vi "Value_Selection_in_Table_GUI.vi"(9 "Column Headers":string[](array[string]), 11 "SELECTION TABLE - Click on values to keep":string[][](table)) -> (2 "Coordinate Array":i32[][](array[numeric]))   [LabVIEW 2020]
uses:
  <vilib>/Utility/miscctls.llb/LVRowAndColumnTypeDef.ctl
  405f9b96-5d72-4015-90c1-6a1ff41fe83b.vi
panel:
  in  "RESET":bool
  in  "DONE":bool
  # "How to use :\n1. The green values are kept\n2. Click the ECS cell if you want to keep the ECS Value.\n2. Reclick the ECS cell if you want to revert to preset value"
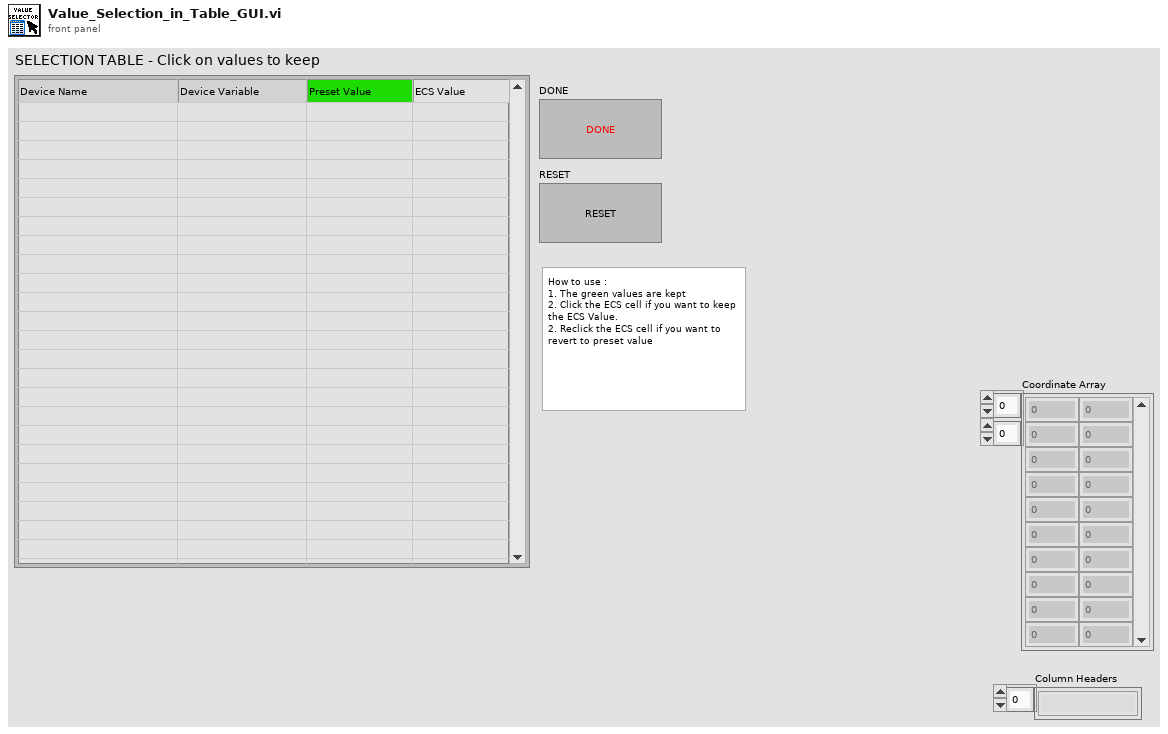
[diagram p1: front panel]
types:
  T1 = typedef "LVRowAndColumnTypeDef.ctl" = cluster{"Row":i32, "Column":i32}
  T2 = typedef "LVPoint32TypeDef.ctl" = cluster{"Horizontal":i32, "Vertical":i32}
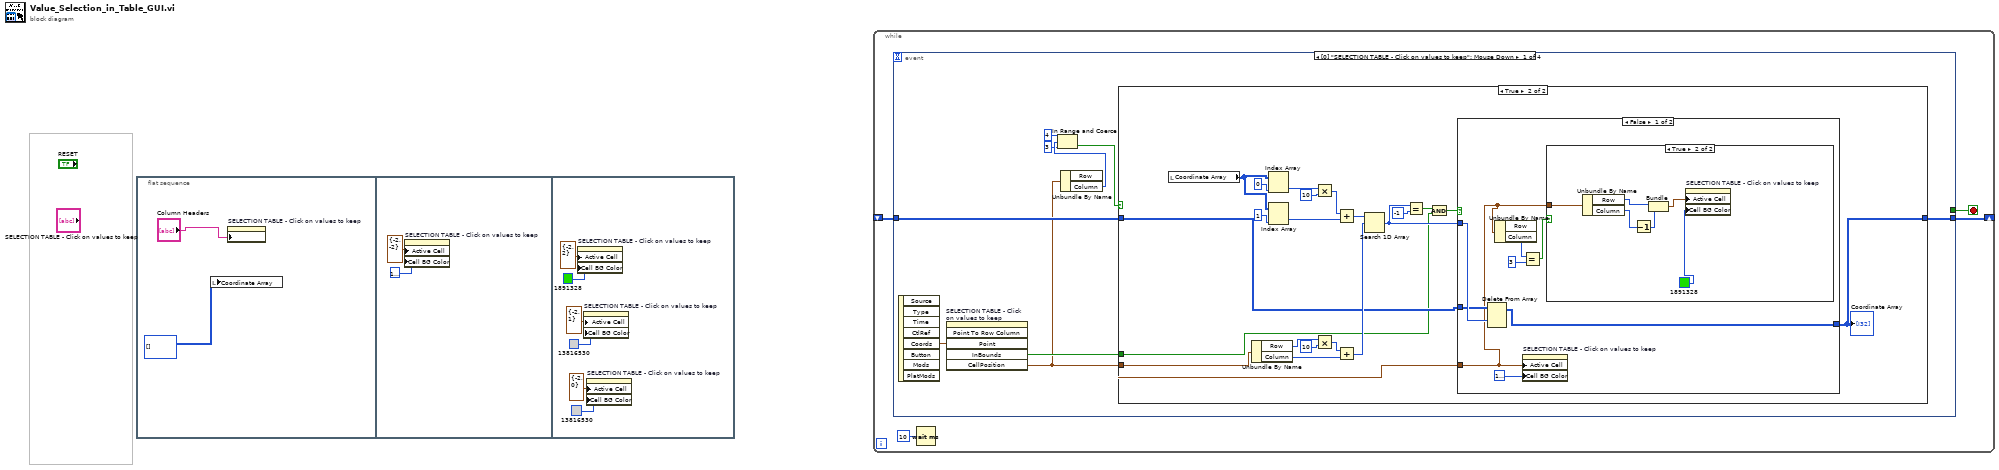
[diagram p0: block diagram]
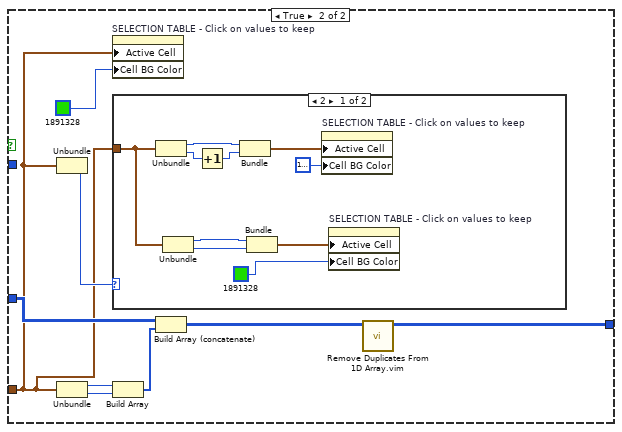
[diagram p4: hidden frame]
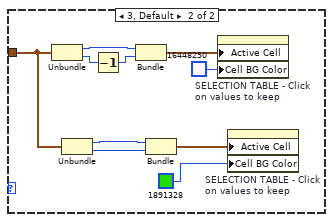
[diagram p5: hidden frame]
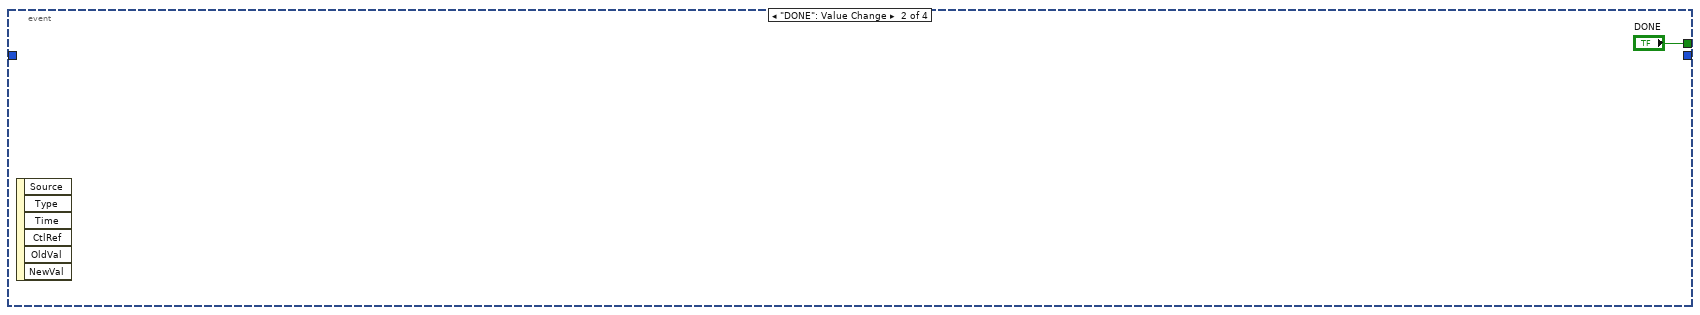
[diagram p6: hidden frame]
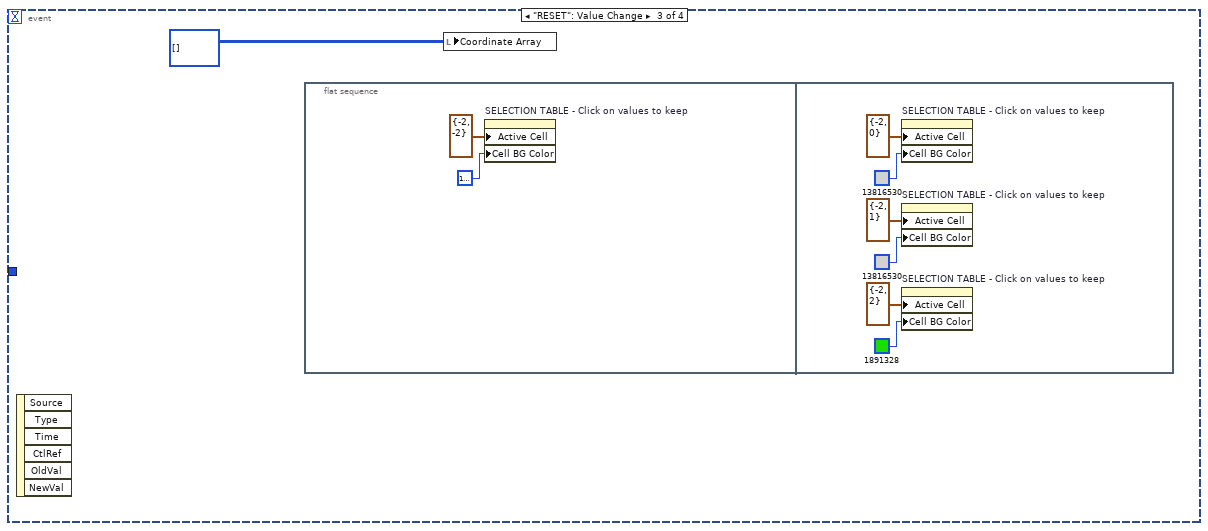
[diagram p7: hidden frame]
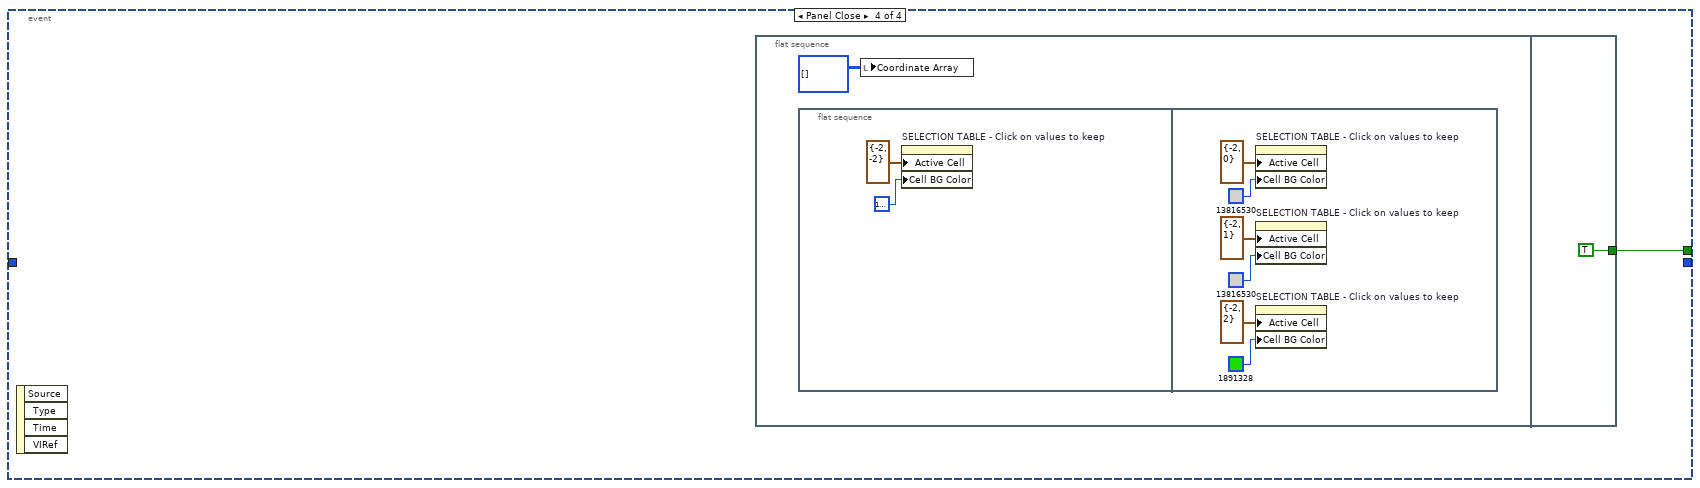
[diagram p8: hidden frame]
diagram:
  n1 = flat-sequence {
    frame #0 {
      n2 = local write "Coordinate Array"(i32[][] []) -> ()
      n3 = property on="SELECTION TABLE - Click on values to keep" class="Tbl (strict)"("Column Headers[]"="Column Headers") -> ()  [unwired: 2 in, 2 out]
    }
    frame #1 {
      n4 = property on="SELECTION TABLE - Click on values to keep" class="Tbl (strict)"("Active Cell"=T1 {"Row"=-2, "Column"=-2} ("Active Cell:Active Cell"), "Cell BG Color"=u32 16777225 ("Active Cell:Cell Background Color")) -> ()  [unwired: 2 in, 2 out]
    }
    frame #2 {
      n5 = property on="SELECTION TABLE - Click on values to keep" class="Tbl (strict)"("Active Cell"=T1 {"Row"=-2, "Column"=2} ("Active Cell:Active Cell"), "Cell BG Color"=u32 1891328 ("Active Cell:Cell Background Color")) -> ()  [unwired: 2 in, 2 out]
      n6 = property on="SELECTION TABLE - Click on values to keep" class="Tbl (strict)"("Active Cell"=T1 {"Row"=-2, "Column"=1} ("Active Cell:Active Cell"), "Cell BG Color"=u32 13816530 ("Active Cell:Cell Background Color")) -> ()  [unwired: 2 in, 2 out]
      n7 = property on="SELECTION TABLE - Click on values to keep" class="Tbl (strict)"("Active Cell"=T1 {"Row"=-2, "Column"=0} ("Active Cell:Active Cell"), "Cell BG Color"=u32 13816530 ("Active Cell:Cell Background Color")) -> ()  [unwired: 2 in, 2 out]
    }
  }
  n8 = while {
    shift-right: [w14] -> _
    shift-left: _ -> [w13]
    stop <- w11 stop-if-true
    n9 = event shown="[0] \"SELECTION TABLE - Click on values to keep\": Mouse Down" {
      selector: _ -> [_ _ _ _]
      dyn-events: _ -> [_ _ _ _]
      timeout: _ -> [_ _ _ _]
      tunnel: [w21 _ _ _] -> w14
      tunnel: w13 -> [w22 _ _ _]
      tunnel: [_ "DONE" _ w99] -> w11
      event "SELECTION TABLE - Click on values to keep": Mouse Down {
        n10 = event-data() -> ("Coords"=w23:T2)  [unwired: 1 in, 7 out]
        n11 = invoke on="SELECTION TABLE - Click on values to keep" class="Tbl (strict)" method="Point To Row Column"("Point"=w23) -> ("InBounds"=w20:bool, "CellPosition"=w19:T1)  [unwired: 5 in, 4 out]
        n12 = Unbundle By Name(w19) -> ("Column"=w17:i32)  [unwired: 1 out]
        n13 = In Range and Coerce(upper limit=4, x=w17, lower limit=3) -> (In Range?=w18:bool)  [unwired: 1 out]
        n14 = case shown="True" w18 {
          tunnel: w19 -> [_ w45]
          tunnel: w22 -> [w24 w30]
          tunnel: [w24 w29] -> w21
          tunnel: w20 -> [_ w25]
          frame False {
          }
          frame True {
            n15 = local read "Coordinate Array"() -> (w36:i32[][])
            n16 = Unbundle By Name(w45) -> ("Row"=w44:i32, "Column"=w42:i32)
            n17 = Index Array(array=w36, index (col)=0 ("index")) -> (element=w38:i32[])  [unwired: 1 in]
            n18 = Index Array(array=w36, index (col)=1 ("index")) -> (element=w34:i32[])  [unwired: 1 in]
            n19 = Multiply(x=w38, y=10) -> (x*y=w40:i32[])
            n20 = Multiply(x=w44, y=10) -> (x*y=w39:i32)
            n21 = Add(x=w40, y=w34) -> (x+y=w33:i32[])
            n22 = Add(x=w39, y=w42) -> (x+y=w32:i32)
            n23 = Search 1D Array(1D array=w33, element=w32) -> (index of element=w28:i32)  [unwired: 1 in]
            n24 = Equal?(x=w28, y=-1) -> (x = y?=w27:bool)
            n25 = And(x=w27, y=w25) -> (x .and. y?=w26:bool)
            n26 = case shown="False" w26 {
              tunnel: w45 -> [w49 w61]
              tunnel: w30 -> [w51 w65]
              tunnel: [w50 w63] -> w29
              tunnel: w28 -> [w52 _]
              frame False {
                n27 = Delete From Array(array=w51, index (row)=w52) -> (array with subset deleted=w50:i32[][])  [unwired: 2 in, 1 out]
                n28 = Unbundle By Name(w49) -> ("Column"=w48:i32)  [unwired: 1 out]
                n29 = Equal?(x=w48, y=3) -> (x = y?=w47:bool)
                n30 = property on="SELECTION TABLE - Click on values to keep" class="Tbl (strict)"("Active Cell"=w49, "Cell BG Color"=u32 16777225 ("Active Cell:Cell Background Color")) -> ()  [unwired: 2 in, 2 out]
                n31 = case shown="True" w47 {
                  tunnel: w49 -> [_ w59]
                  frame False {
                  }
                  frame True {
                    n32 = Unbundle By Name(w59) -> ("Row"=w58:i32, "Column"=w56:i32)
                    n33 = Decrement(x=w56) -> (x-1=w55:i32)
                    n34 = Bundle("Row"=w58, w55) -> (w57:cluster{"Row":i32, i32})  [unwired: 1 in]
                    n35 = property on="SELECTION TABLE - Click on values to keep" class="Tbl (strict)"("Active Cell"=w57, "Cell BG Color"=u32 1891328 ("Active Cell:Cell Background Color")) -> ()  [unwired: 2 in, 2 out]
                  }
                }
              }
              frame True {
                n36 = Unbundle(w61) -> ("Column"=w62:i32)  [unwired: 1 out]
                n37 = Unbundle(w61) -> ("Row"=w66:i32, "Column"=w67:i32)
                n38 = property on="SELECTION TABLE - Click on values to keep" class="Tbl (strict)"("Active Cell"=w61, "Cell BG Color"=u32 1891328 ("Active Cell:Cell Background Color")) -> ()  [unwired: 2 in, 2 out]
                n39 = case shown="2" w62 {
                  tunnel: w61 -> [w71 w81]
                  frame 2 {
                    n40 = Unbundle(w71) -> ("Row"=w74:i32, "Column"=w77:i32)
                    n41 = Unbundle(w71) -> ("Row"=w73:i32, "Column"=w70:i32)
                    n42 = Increment(x=w77) -> (x+1=w75:i32)
                    n43 = Bundle("Row"=w74, w75) -> (w76:cluster{"Row":i32, i32})  [unwired: 1 in]
                    n44 = Bundle("Row"=w73, "Column"=w70) -> (w72:cluster{"Row":i32, "Column":i32})  [unwired: 1 in]
                    n45 = property on="SELECTION TABLE - Click on values to keep" class="Tbl (strict)"("Active Cell"=w76, "Cell BG Color"=u32 16777225 ("Active Cell:Cell Background Color")) -> ()  [unwired: 2 in, 2 out]
                    n46 = property on="SELECTION TABLE - Click on values to keep" class="Tbl (strict)"("Active Cell"=w72, "Cell BG Color"=u32 1891328 ("Active Cell:Cell Background Color")) -> ()  [unwired: 2 in, 2 out]
                  }
                  frame 3, Default {
                    n47 = Unbundle(w81) -> ("Row"=w84:i32, "Column"=w87:i32)
                    n48 = Unbundle(w81) -> ("Row"=w83:i32, "Column"=w80:i32)
                    n49 = Decrement(x=w87) -> (x-1=w85:i32)
                    n50 = Bundle("Row"=w84, w85) -> (w86:cluster{"Row":i32, i32})  [unwired: 1 in]
                    n51 = Bundle("Row"=w83, "Column"=w80) -> (w82:cluster{"Row":i32, "Column":i32})  [unwired: 1 in]
                    n52 = property on="SELECTION TABLE - Click on values to keep" class="Tbl (strict)"("Active Cell"=w86, "Cell BG Color"=u32 16448250 ("Active Cell:Cell Background Color")) -> ()  [unwired: 2 in, 2 out]
                    n53 = property on="SELECTION TABLE - Click on values to keep" class="Tbl (strict)"("Active Cell"=w82, "Cell BG Color"=u32 1891328 ("Active Cell:Cell Background Color")) -> ()  [unwired: 2 in, 2 out]
                  }
                }
                n54 = Build Array(w66, w67) -> (w68:i32[])
                n55 = Build Array (concatenate)(w65, w68) -> (w64:i32[][])
                n56 = call "Remove Duplicates From 1D Array.vim"("array"=w64) -> ("array with duplicates removed"=w63:i32[][])  [unwired: 10 in]
              }
            }
            "Coordinate Array" <- w29
          }
        }
      }
      event "DONE": Value Change {
        n57 = event-data() -> ()  [unwired: 1 in, 6 out]
      }
      event "RESET": Value Change {
        n58 = event-data() -> ()  [unwired: 1 in, 6 out]
        n59 = flat-sequence {
          frame #0 {
            n60 = property on="SELECTION TABLE - Click on values to keep" class="Tbl (strict)"("Active Cell"=T1 {"Row"=-2, "Column"=-2} ("Active Cell:Active Cell"), "Cell BG Color"=u32 16777225 ("Active Cell:Cell Background Color")) -> ()  [unwired: 2 in, 2 out]
          }
          frame #1 {
            n61 = property on="SELECTION TABLE - Click on values to keep" class="Tbl (strict)"("Active Cell"=T1 {"Row"=-2, "Column"=0} ("Active Cell:Active Cell"), "Cell BG Color"=u32 13816530 ("Active Cell:Cell Background Color")) -> ()  [unwired: 2 in, 2 out]
            n62 = property on="SELECTION TABLE - Click on values to keep" class="Tbl (strict)"("Active Cell"=T1 {"Row"=-2, "Column"=1} ("Active Cell:Active Cell"), "Cell BG Color"=u32 13816530 ("Active Cell:Cell Background Color")) -> ()  [unwired: 2 in, 2 out]
            n63 = property on="SELECTION TABLE - Click on values to keep" class="Tbl (strict)"("Active Cell"=T1 {"Row"=-2, "Column"=2} ("Active Cell:Active Cell"), "Cell BG Color"=u32 1891328 ("Active Cell:Cell Background Color")) -> ()  [unwired: 2 in, 2 out]
          }
        }
        n64 = local write "Coordinate Array"(i32[][] []) -> ()
      }
      event Panel Close {
        n65 = event-data() -> ()  [unwired: 1 in, 4 out]
        n66 = flat-sequence {
          tunnel: [TRUE] -> w99
          frame #0 {
            n67 = flat-sequence {
              frame #0 {
                n68 = property on="SELECTION TABLE - Click on values to keep" class="Tbl (strict)"("Active Cell"=T1 {"Row"=-2, "Column"=-2} ("Active Cell:Active Cell"), "Cell BG Color"=u32 16777225 ("Active Cell:Cell Background Color")) -> ()  [unwired: 2 in, 2 out]
              }
              frame #1 {
                n69 = property on="SELECTION TABLE - Click on values to keep" class="Tbl (strict)"("Active Cell"=T1 {"Row"=-2, "Column"=0} ("Active Cell:Active Cell"), "Cell BG Color"=u32 13816530 ("Active Cell:Cell Background Color")) -> ()  [unwired: 2 in, 2 out]
                n70 = property on="SELECTION TABLE - Click on values to keep" class="Tbl (strict)"("Active Cell"=T1 {"Row"=-2, "Column"=1} ("Active Cell:Active Cell"), "Cell BG Color"=u32 13816530 ("Active Cell:Cell Background Color")) -> ()  [unwired: 2 in, 2 out]
                n71 = property on="SELECTION TABLE - Click on values to keep" class="Tbl (strict)"("Active Cell"=T1 {"Row"=-2, "Column"=2} ("Active Cell:Active Cell"), "Cell BG Color"=u32 1891328 ("Active Cell:Cell Background Color")) -> ()  [unwired: 2 in, 2 out]
              }
            }
            n72 = local write "Coordinate Array"(i32[][] []) -> ()
          }
          frame #1 {
          }
        }
      }
    }
    n73 = Wait (ms)(milliseconds to wait=u32 10) -> ()  [unwired: 1 out]
  }
